vi "Find Class Path.vi"(7 "basepath":path, 8 "error in (no error)":errorcluster, 11 "Configuration in":refnum<class "Configuration.lvclass">) -> (0 "error out":errorcluster, 1 "LegalClass":bool, 2 "Class Path":path, 3 "Configuration out":refnum<class "Configuration.lvclass">)   [LabVIEW 2023, in "Configuration.lvlib" / "Configuration.lvclass"]
uses:
  Library/Configuration.lvclass
  Library/Configuration.lvclass/Configuration.ctl
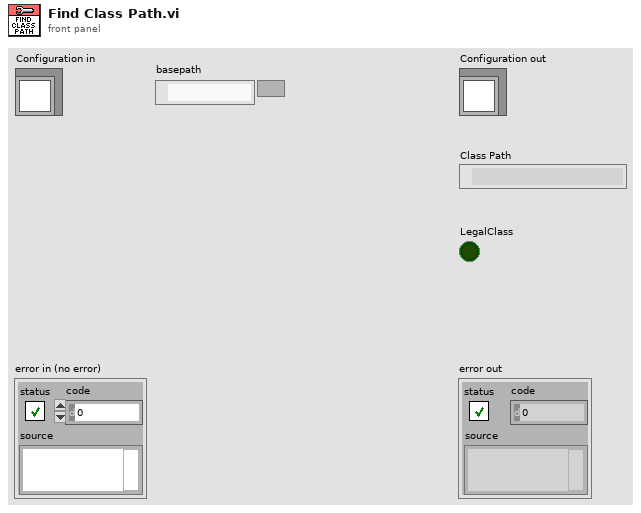
[diagram p1: front panel]
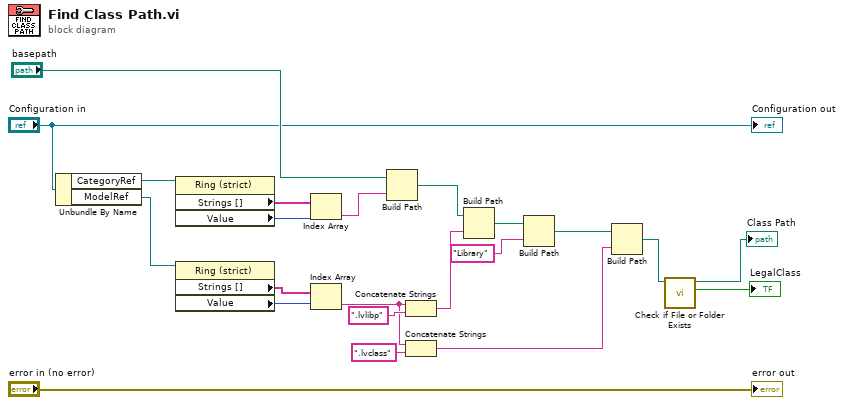
[diagram p0: block diagram]
diagram:
  n1 = Unbundle By Name("Configuration in") -> ("CategoryRef"=w22:refnum<vi>, "ModelRef"=w21:refnum<vi>)
  n2 = property class="Ring (strict)"(reference=w22) -> ("Strings []"=w20:string[], "Value"=w19:u16)  [unwired: 1 in, 2 out]
  n3 = property class="Ring (strict)"(reference=w21) -> ("Strings []"=w18:string[], "Value"=w17:u16)  [unwired: 1 in, 2 out]
  n4 = Index Array(array=w20, index=w19) -> (element=w16:string)
  n5 = Index Array(array=w18, index=w17) -> (element=w7:string)
  n6 = Build Path(base path="basepath", name or relative path=w16) -> (appended path=w11:path)
  n7 = Concatenate Strings(w7, ".lvlibp" ("regular expression")) -> (w8:string)
  n8 = Concatenate Strings(w7, ".lvclass" ("string")) -> (w4:string)
  n9 = Build Path(base path=w11, name or relative path=w8) -> (appended path=w10:path)
  n10 = Build Path(base path=w10, name or relative path="Library" ("regular expression")) -> (appended path=w5:path)
  n11 = Build Path(base path=w5, name or relative path=w4) -> (appended path=w3:path)
  n12 = call <vilib>:"Check if File or Folder Exists.vi"("path"=w3) -> ("file or folder exists?"=→"LegalClass":bool, "dup path"=→"Class Path":path)  [unwired: 8 in, 1 out]
  "error out" <- "error in (no error)"
  "Configuration out" <- "Configuration in"
